vi "Single Motor Control.vi"() -> ()   [LabVIEW 2017]
doc: "<B>Motor Control.vi</B> demonstrates simplistic control of a motor using PWM.\n\nThis example expects a USB cable connected from your development PC to the Type B USB Jack (next to the power input) on the roboRIO.\n\nThis example requires the Driver Station to be running with Teleoperated Enabled."
uses:
  <vilib>/Rock Robotics/SystemInterfaces/DIO/FPGA_DIOPWMChannel.ctl
  <vilib>/Rock Robotics/WPI/MotorControl/WPI_MotorControlOpen SPARK.vi
panel:
  in  "Speed (-1 to 1)":dbl(slide) min=-1.0 max=1.0 step=0.1 scale=-1.0..1.0 scale format="%#.3f"
  in  "PWM Channel":T1
  in  "stop":bool
  # "Set this input before running."
  # "This can be set while running."
  # "This example requires the Driver Station to be running with Teleoperated Enabled."
  # "PWM cable"
  # "This shows wiring for a Talon speed controller.  The wiring is similar for Victor and Jaguar controllers.  If you change the controller type, you must also select the appropriate instance of the Motor Open VI on the diagram."
  # "Power\nTerminals"
  # "Motor\nTerminals"
  # "+"
  # "+"
  # "M"
  # "B"
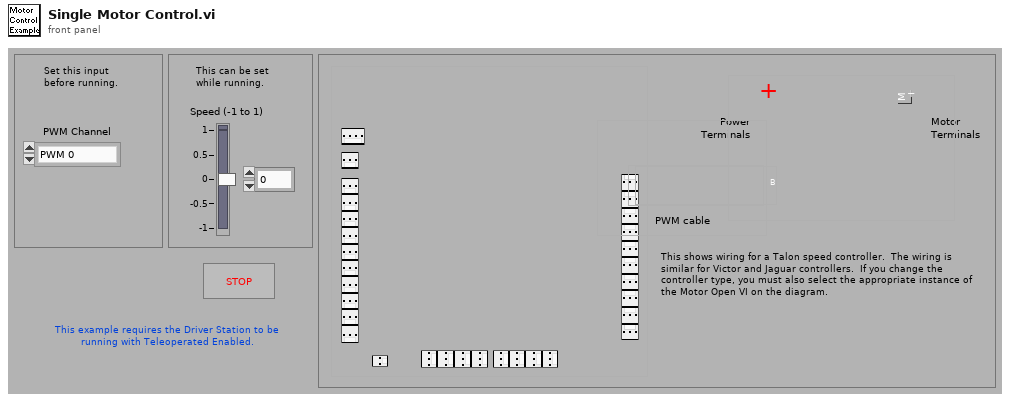
[diagram p1: front panel]
types:
  T1 = typedef "FPGA_DIOPWMChannel.ctl" = enum8{"PWM 0", "PWM 1", "PWM 2", "PWM 3", "PWM 4", "PWM 5", "PWM 6", "PWM 7", "PWM 8", "PWM 9", "PWM MXP 0", "PWM MXP 1", "PWM MXP 2", "PWM MXP 3", "PWM MXP 4", "PWM MXP 5", "PWM MXP 6", "PWM MXP 7", "PWM MXP 8", "PWM MXP 9", "Invalid"}
  T2 = typedef "WPI_MotorControlDeviceRef.ctl" = cluster{"DeviceStatus":errorcluster, "Type":T3, "PWM":cluster{"PWM Channel":T1, "DeadBand":T4}, "CAN":cluster{"Device Number":u8, "SetOutput VI Ref":variant, "GetOutput VI Ref":variant, "Enable VI Ref":variant, "Disable VI Ref":variant, "Data":variant}, "Invert":bool, "DIO PWM":cluster{"PWM \"Enable\" Channel":T1, "DIOChannel":T5, "PWM Rate":dbl}}
  T3 = typedef "WPI_MotorControlType.ctl" = enum16{"PWM", "CAN", "DIO PWM"}
  T4 = typedef "WPI_PWMDeadband.ctl" = cluster{"Name":string, "maxPositivePwm":i32, "minPositivePwm":i32, "centerPwm":i32, "maxNegativePwm":i32, "minNegativePwm":i32, "angularRange":u16}
  T5 = typedef "FPGA_DIOChannel.ctl" = enum8{"DIO 0", "DIO 1", "DIO 2", "DIO 3", "DIO 4", "DIO 5", "DIO 6", "DIO 7", "DIO 8", "DIO 9", "DIO MXP 0", "DIO MXP 1", "DIO MXP 2", "DIO MXP 3", "DIO MXP 4", "DIO MXP 5", "DIO MXP 6", "DIO MXP 7", "DIO MXP 8", "DIO MXP 9", "DIO MXP 10", "DIO MXP 11", "DIO MXP 12", "DIO MXP 13", "DIO MXP 14", "DIO MXP 15", "SPI Port CS1", "SPI Port CS2", "SPI Port CS3", "SPI Port MISO", "SPI Port MOSI", "Invalid"}
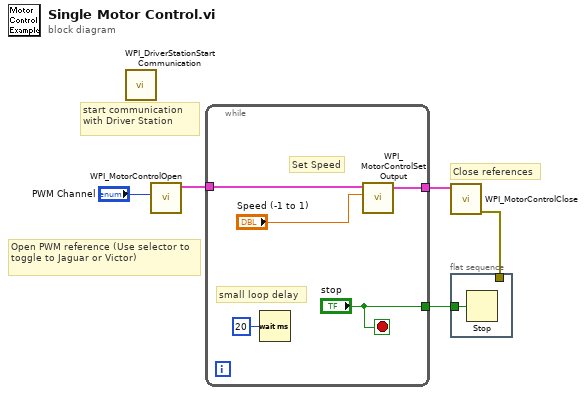
[diagram p0: block diagram]
diagram:
  # "start communication with Driver Station"
  # "Close references"
  # "Open PWM reference (Use selector to toggle to Jaguar or Victor)"
  n1 = call <vilib>:"WPI_DriverStationStart Communication.vi"() -> ()  [unwired: 2 in, 10 out]
  n2 = call-poly <vilib>:"WPI_MotorControlOpen.vi"("PWM Channel"="PWM Channel") -> ("MotorControlDeviceRef"=w4:T2)  [unwired: 3 in, 7 out]
  n3 = while {
    tunnel: w4 -> [w10]
    tunnel: [w8] -> w3
    tunnel: ["stop"] -> w2
    stop <- "stop" stop-if-true
    # "small loop delay"
    # "Set Speed"
    n4 = Wait (ms)(milliseconds to wait=u32 20) -> ()  [unwired: 1 out]
    n5 = call <vilib>:"WPI_MotorControlSetOutput.vi"("Output"="Speed (-1 to 1)", "MotorControlDevRef"=w10) -> ("MotorControlDevRef"=w8:T2)  [unwired: 2 in, 7 out]
  }
  n6 = call <vilib>:"WPI_MotorControlClose.vi"("MotorControlDevRef"=w3) -> ("error out"=w1:errorcluster)  [unwired: 1 in, 9 out]
  n7 = flat-sequence {
    tunnel: w2 -> [w11]
    tunnel: w1 -> [_]
    frame #0 {
      n8 = Stop(stop? (T)=w11) -> ()
    }
  }
